vi "Update Record Length based on Trig Offset.vi"(8 "Start of Record":bool=TRUE, 10 "Points to Acquire":u16, 11 "Trigger Offset":u8) -> (2 "Updated Points to Acquire":u16)   [LabVIEW 2011]
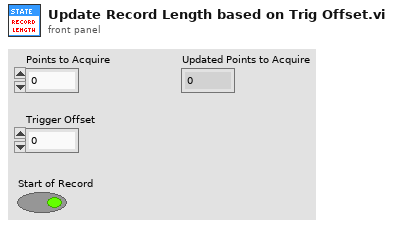
[diagram p1: front panel]
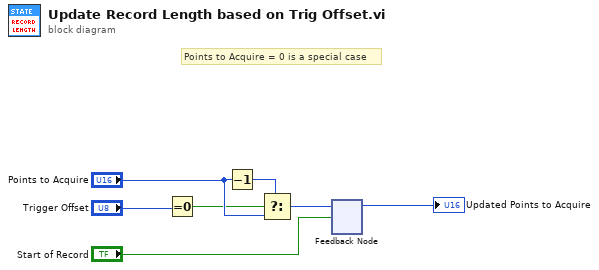
[diagram p0: block diagram]
diagram:
  # "Points to Acquire = 0 is a special case"
  n1 = Equal To 0?(x="Trigger Offset") -> (x = 0?=w4:bool)
  n2 = Decrement(x="Points to Acquire") -> (x-1=w7:u16)
  n3 = Select(t=w7, s=w4, f="Points to Acquire") -> (s? t:f=w5:u16)
  n4 = feedback-in #1(w5, "Start of Record") -> ()
  n5 = feedback #1() -> (→"Updated Points to Acquire":u16)  [unwired: 1 in]
